vi "Initialize Sessions.vi"   [LabVIEW 2020, in "Plug-In SDK VISA Sessions.lvlib"]
doc: "Create the VISA session(s) from the <b>session reservation in</b> and the <b>instrument type id</b>. The <b>instrument type id</b> must match the Instrument Type Id for the custom VISA instrument in the pin map."
uses:
  Plug-In SDK VISA Sessions.lvlib
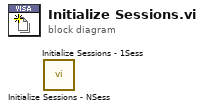
[diagram p0: block diagram]
diagram:
  n1 = call "Initialize Sessions - NSess.vi"() -> ()  [unwired: 8 in, 4 out]
  n2 = call "Initialize Sessions - 1Sess.vi"() -> ()  [unwired: 8 in, 4 out]
